vi "Init Hardware.vi"(8 "error in (no error)":errorcluster, 11 "Red Pitaya Lock-in Driver in":refnum<class "Red Pitaya Lock-in Driver.lvclass">) -> (0 "error out":errorcluster, 3 "Red Pitaya Lock-in Driver out":refnum<class "Red Pitaya Lock-in Driver.lvclass">)   [LabVIEW 2016, in "Red Pitaya Lock-in Driver.lvclass"]
uses:
  Red Pitaya Lock-in Driver.lvclass
  C:/github/NHMFL_Core/Libraries/Instruments/Instrument Driver/Lock-in Driver/Lock-in Driver.lvclass
  C:/github/NHMFL_Core/Libraries/Instruments/Instrument Driver/Instrument Driver.lvclass
  Red Pitaya Lock-in Driver.lvclass/Red Pitaya Lock-in Driver.ctl
  Instruments/Instrument Driver/Instrument Driver.lvclass/Instrument Driver.ctl
  RP Instrument/RP Instrument.lvclass/RP Instrument.ctl
  Read RP Instrument.vi
  Instruments/Instrument Driver/Read Recorder name.vi
  RP Instrument/Write Decimation.vi
  Write RP Instrument.vi
  Instruments/Instrument Driver/Write Channel names.vi
  Instruments/Instrument Driver/Lock-in Driver/Read Lock-in configuration.vi
  RP Instrument/RP Instrument.lvclass
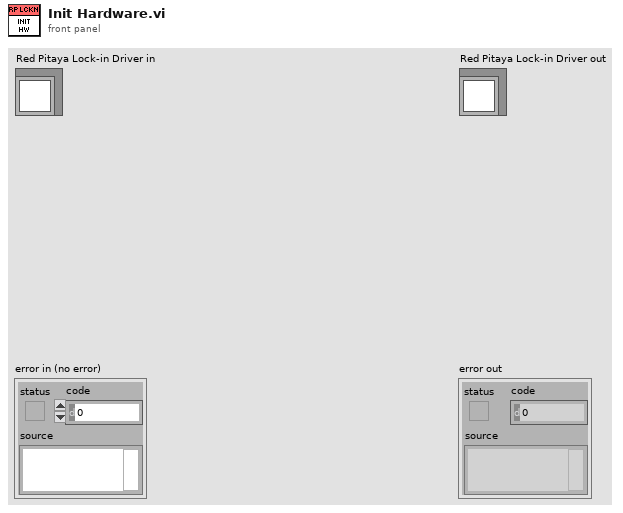
[diagram p1: front panel]
types:
  T1 = typedef "Lock-in Configuration.ctl" = cluster{"Frequency":dbl, "Time constant":dbl, "Synchronous":bool, "Channels":i32[]}
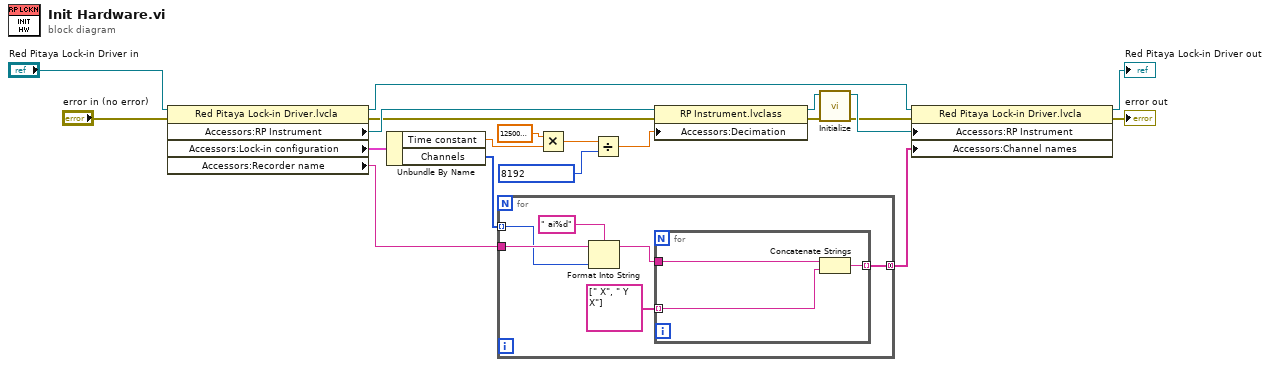
[diagram p0: block diagram]
diagram:
  n1 = property class="Red Pitaya Lock-in Driver.lvcla"(reference="Red Pitaya Lock-in Driver in", error in="error in (no error)") -> (reference out=w18:refnum<class "Red Pitaya Lock-in Driver.lvclass">, error out=w12:errorcluster, "Accessors:RP Instrument"=w19:refnum<class "RP Instrument.lvclass">, "Accessors:Lock-in configuration"=w11:T1, "Accessors:Recorder name"=w2:string)
  n2 = Unbundle By Name(w11) -> ("Time constant"=w9:dbl, "Channels"=w3:i32[])
  n3 = for {
    tunnel: w3 -> [w21] mode=indexing
    tunnel: w2 -> [w25]
    tunnel: [w22] -> w1 mode=concatenating
    n4 = Format Into String(format string=" ai%d", initial string=w25, w21) -> (resulting string=w23:string)  [unwired: 1 in, 1 out]
    n5 = for {
      tunnel: string[] [" X", " Y X"] -> [w29] mode=indexing
      tunnel: w23 -> [w28]
      tunnel: [w27] -> w22 mode=indexing
      n6 = Concatenate Strings(w28, w29) -> (w27:string)
    }
  }
  n7 = Multiply(x=125000000.0, y=w9) -> (x*y=w8:dbl)
  n8 = Divide(x=w8, y=u32 8192 ("IDN response")) -> (x/y=w6:dbl)
  n9 = property class="RP Instrument.lvclass"(reference=w19, error in=w12, "Accessors:Decimation"=w6) -> (reference out=w13:refnum<class "RP Instrument.lvclass">, error out=w5:errorcluster)
  n10 = call-dynamic "Initialize.vi"("error in (no error)"=w5, "RP Instrument in"=w13) -> ("error out"=w4:errorcluster, "RP Instrument out"=w17:refnum<class "RP Instrument.lvclass">)  [unwired: 8 in]
  n11 = property class="Red Pitaya Lock-in Driver.lvcla"(reference=w18, error in=w4, "Accessors:RP Instrument"=w17, "Accessors:Channel names"=w1) -> (reference out=→"Red Pitaya Lock-in Driver out":refnum<class "Red Pitaya Lock-in Driver.lvclass">, error out=→"error out":errorcluster)
